vi "WSVCAP SHL Host TL SPI Write_Read - Single DUT.vi"(0 "Data Out":string, 11 "error in":errorcluster, 12 "Log (T)":bool=TRUE, 13 "DUT":T1) -> (4 "Data In":string, 15 "error out":errorcluster)   [LabVIEW 2012]
uses:
  Type Defs/WSVCAP SHL DUT Number Enum.ctl
panel:
  out "SPI Data In":u8[][](array[numeric]) format="%02x"
  out "Socket Mask":u16=1 format="%02x"
  out "SPI Data Out":u8[][](array[numeric]) format="%02x"
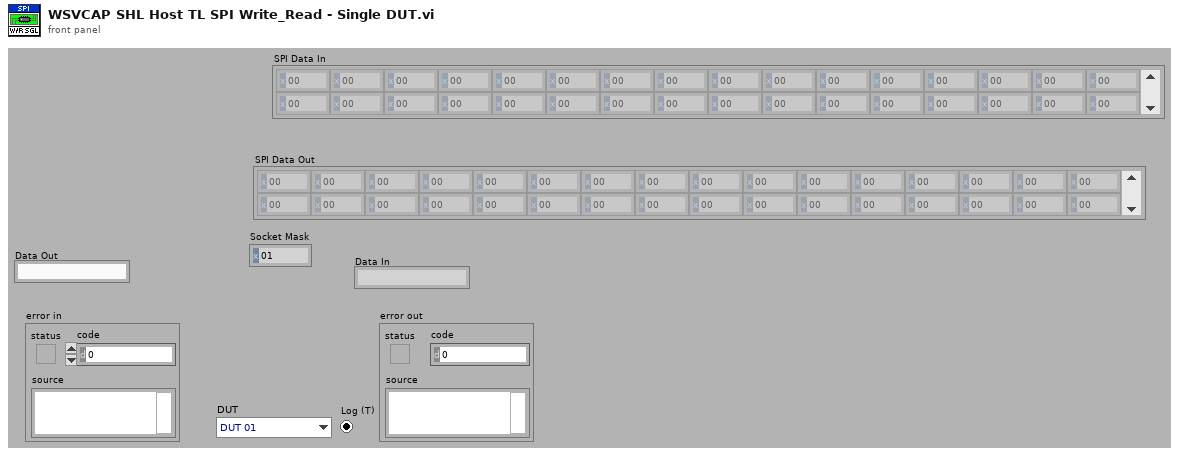
[diagram p1: front panel]
types:
  T1 = typedef "WSVCAP SHL DUT Number Enum.ctl" = enum16{"DUT 01", "DUT 02", "DUT 03", "DUT 04", "DUT 05", "DUT 06", "DUT 07", "DUT 08", "DUT 09", "DUT 10", "DUT 11", "DUT 12", "DUT 13", "DUT 14", "DUT 15", "DUT 16", "DUT 17", "DUT 18", "DUT 19", "DUT 20", "DUT 21", "DUT 22", "DUT 23", "DUT 24", "DUT 25", "DUT 26", "DUT 27", "DUT 28", "DUT 29", "DUT 30", "DUT 31", "DUT 32", "DUT 33", "DUT 34", "DUT 35", "DUT 36"}
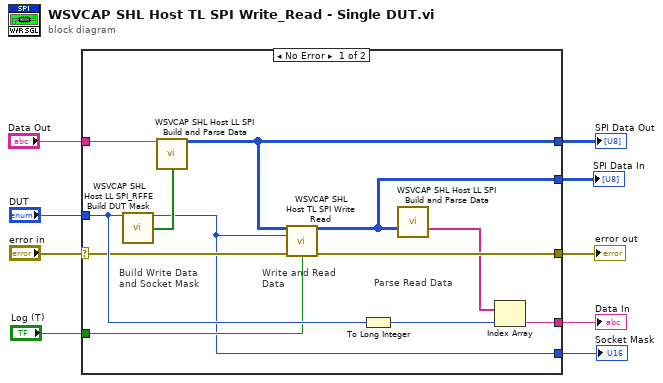
[diagram p0: block diagram]
diagram:
  n1 = case shown="No Error" "error in" {
    selector: "error in" -> [w20 _]
    tunnel: [w19 _] -> w9
    tunnel: "Data Out" -> [w18 _]
    tunnel: [w16 _] -> w6
    tunnel: "DUT" -> [w21 _]
    tunnel: [w14 _] -> w4
    tunnel: [w12 _] -> w3
    tunnel: [w10 _] -> w2
    tunnel: "Log (T)" -> [w13 _]
    frame No Error {
      # "Parse Read Data"
      # "Write and Read\nData"
      # "Build Write Data and Socket Mask"
      n2 = call "WSVCAP SHL Host LL SPI_RFFE Build DUT Mask.vi"("DUT"=w21) -> ("Socket Mask [U64]"=w12:u64, "DUT Mask"=w17:bool[])  [unwired: 13 in]
      n3 = call "WSVCAP SHL Host LL SPI Build and Parse Data.vi"("Data Out"=w18, "DUT Mask (All)"=w17) -> ("SPI Data Out [U8]"=w16:u8[][])  [unwired: 10 in, 3 out]
      n4 = call "WSVCAP SHL Host TL SPI Write Read.vi"("SPI Data Out"=w16, "Socket Mask"=w12, "error in"=w20, "Log (T)"=w13) -> ("Read Data Out"=w10:u8[][], "error out"=w19:errorcluster)  [unwired: 10 in]
      n5 = To Long Integer(number=w21) -> (32bit integer=w15:i32)
      n6 = call "WSVCAP SHL Host LL SPI Build and Parse Data.vi"("SPI Data In [U8]"=w10) -> ("SPI Data In"=w11:string[])  [unwired: 11 in, 3 out]
      n7 = Index Array(array=w11, index=w15) -> (element=w14:string)
    }
    frame Error {
    }
  }
  "error out" <- w9
  "SPI Data Out" <- w6
  "Socket Mask" <- w3
  "Data In" <- w4
  "SPI Data In" <- w2
